vi "GetProbePlanCoordinates.vi"(1 "Probe Card Channels":i32=32) -> (0 "file path":string, 2 "OK?":bool, 3 "Array":T1(array[cluster]))   [LabVIEW 2019]
doc: "Utility to read probe plan from text file and generate respective coordinates in global variable."
uses:
  general_VIs/globals/QC_MeasurementSetup.vi
  ProbePlanParams.vi
  <vilib>/regexp/Match Regular Expression.xnode
panel:
  out "No. probe points":string
  in  "ProbePoints":T2
  out "String":string
  in  "Stop Button":bool
  in  "OK Button":bool
  in  "Region":u16(ring)
  out "Coordinates":string[][](table)
  # "ProbePlan Coordinates"
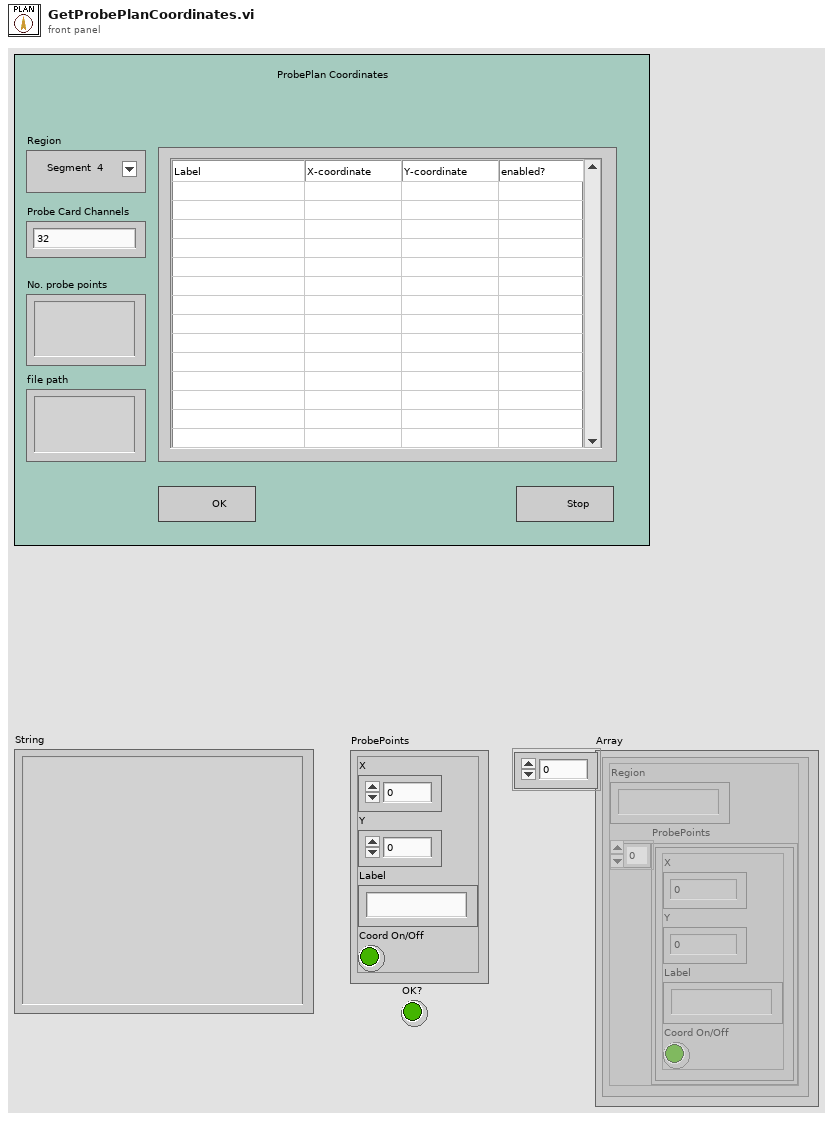
[diagram p1: front panel]
types:
  T1 = cluster{"Region":string, "ProbePoints":cluster{"X":dbl, "Y":dbl, "Label":string, "Coord On/Off":bool}[]}[]
  T2 = cluster{"X":dbl, "Y":dbl, "Label":string, "Coord On/Off":bool}
  T3 = cluster{"Region":string, "ProbePoints":cluster{"X":dbl, "Y":dbl, "Label":string, bool}[]}[]
  T4 = enum16{"open", "replace", "create", "open or create", "replace or create", "replace or create with confirmation"}
  T5 = cluster{"X":dbl, "Y":dbl, "Label":string, bool}[]
  T6 = cluster{"Bias Supply":refnum<class "SupplyControl.lvclass">, "SMU":refnum<class "SupplyControl.lvclass">, "LCR":refnum<class "LCRControl.lvclass">, "Probe Card Channels":i32, "Bias Voltage [V]":dbl, "First strip":i32, "Last strip":i32, "Base Voltage [V]":dbl, "Base Ramp Step [V]":dbl, "Base Ramp Interval [ms]":u32, "High Voltage [V]":dbl, "High Ramp Step [V]":dbl, "High Ramp Interval [ms]":u32, "AC frequency [Hz]":i32, "AC amplitude [V]":dbl, "RC Configuration":u16, "Single Needle":bool, "Temperature Readout":enum16{"Read Arduino", "Enter manually"}, "Arduino":refnum<class "ArduinoControl.lvclass">, "Fraction of good strips [%]":dbl, "ProbeStation":refnum<class "ProbeStationControl.lvclass">, "Switching":refnum<class "Switching.lvclass">, "Matrix used?":bool, "Matrix X Channels":cluster{"Bias Supply / SMU LO":i32, "Bias Supply / SMU HI":i32, "CV Box LO":i32, "CV Box HI":i32, "CV Box LO IN":i32, "CV Box HI IN":i32, "Volt meter LO":i32, "Volt meter HI":i32, "Mux1 C1":i32, "Mux1 C2":i32, "Mux2 C1":i32, "Mux2 C2":i32}, "Pinholes Y/N":bool, "Capacitance Y/N":bool, "Resistance Y/N":bool, "Bias Supply Name":string, "SMU Name":string, "LCR Name":string}
  T7 = cluster{"submatch 1":string, "ProbePoints":cluster{"X":dbl, "Y":dbl, "Label":string, bool}[]}
  T8 = cluster{"submatch 1":string, "ProbePoints":cluster{"X":dbl, "Y":dbl, "Label":string, bool}[]}[]
  T9 = cluster{"Region":string, "ProbePoints":cluster{"X":dbl, "Y":dbl, "Label":string, bool}[]}
  T10 = cluster{"X":dbl, "Y":dbl, "Label":string, "Coord On/Off":bool}[]
  T11 = cluster{"Region":string, cluster{"X":dbl, "Y":dbl, "Label":string, "Coord On/Off":bool}[]}
  T12 = cluster{"Strip Number OUT":i32, "X0":i32, "Y0":i32, "X1":i32, "Y1":i32, "Xref":dbl, "Yref":dbl, "ProbePlan type":u32, "Inner pads offset":ext, "Outer pads offset":ext, "l_inner":ext, "l_outer":ext, "strip numbering":u16, "Device Orientation":ext, "Stagger offset":i32, "Yoffset":dbl, "Strip pitch":dbl, "Fiducail separation":dbl, "Radius":ext, "Relative strip angles":dbl, "Probeplan description":string, "ProbePlan array":cluster{"Region":string, "ProbePoints":cluster{"X":dbl, "Y":dbl, "Label":string, "CardViable?":bool}[]}[], "Test ProbePoints":cluster{"Regions Enabled":bool[], "From index":u32[], "To index":u32[]}}
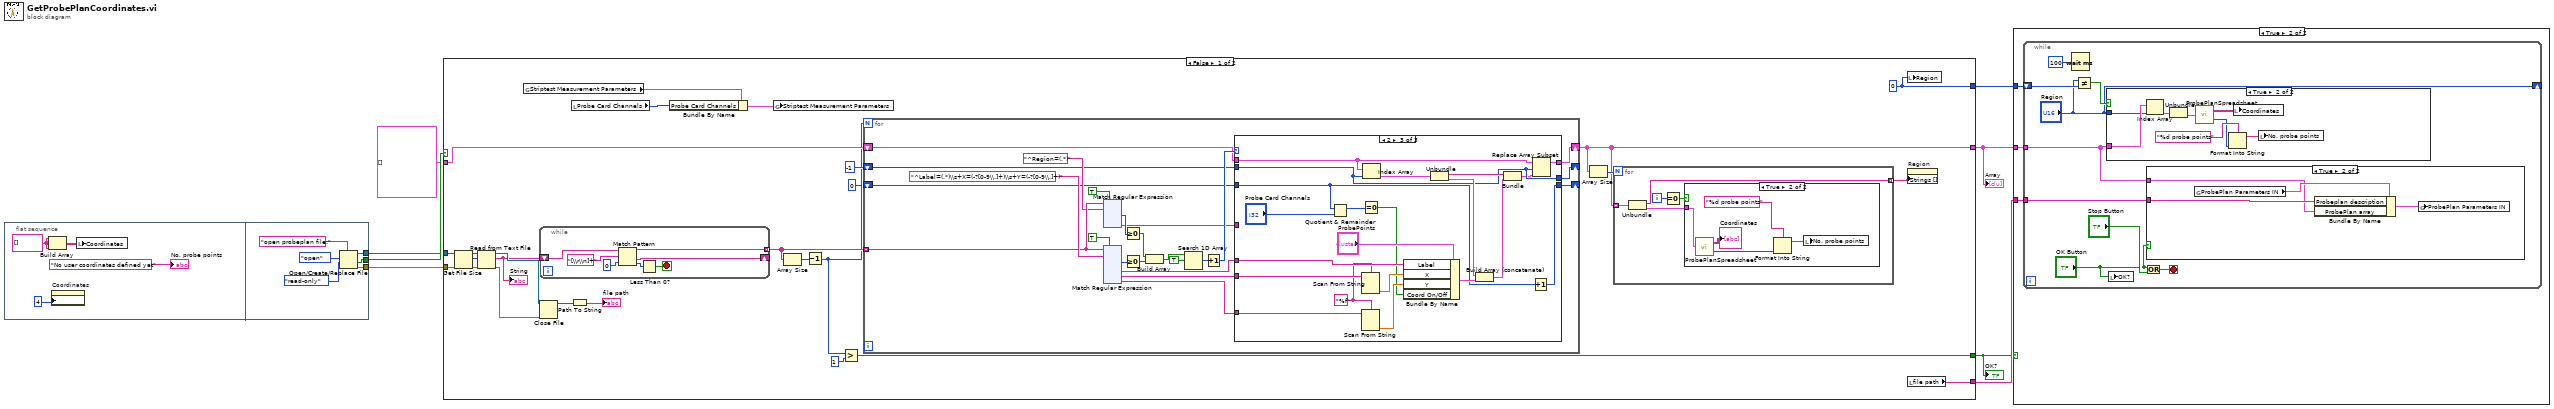
[diagram p0: block diagram]
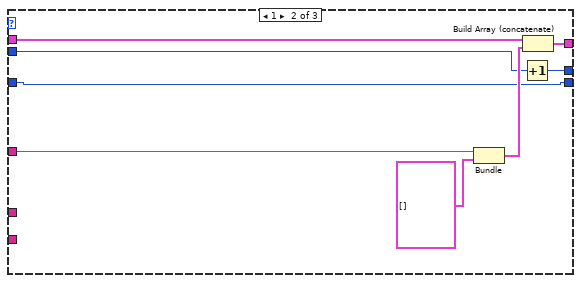
[diagram p7: hidden frame]
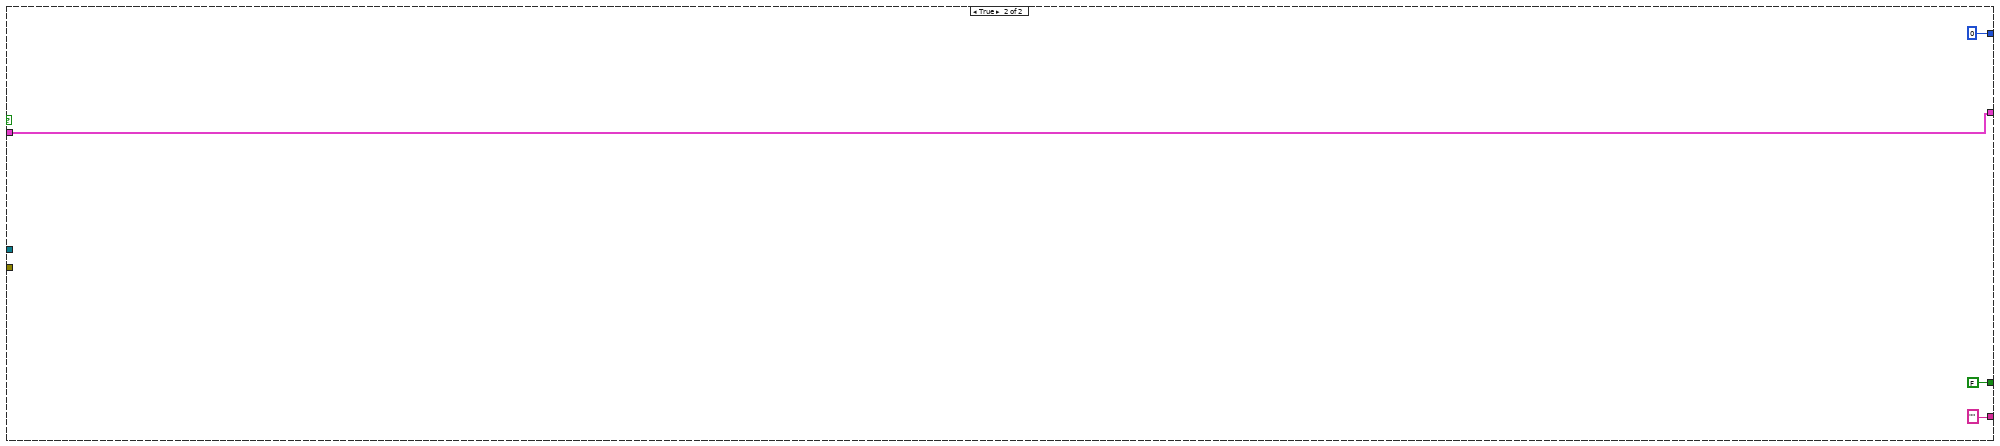
[diagram p8: hidden frame]
diagram:
  n1 = flat-sequence {
    tunnel: [w15] -> w8
    tunnel: [w14] -> w6
    tunnel: [w13] -> w7
    frame #0 {
      w12 = string[] []
      n2 = Build Array(w12, w12, w12) -> (w11:string[][])
      n3 = property on="Coordinates" class="Tbl (strict)"("Number of Columns"=4) -> ()  [unwired: 2 in, 2 out]
      n4 = local write "Coordinates"(w11) -> ()
      "No. probe points" <- "No user coordinates defined yet" ("String 2")
    }
    frame #1 {
      n5 = Open/Create/Replace File(prompt="open probeplan file:", operation (0:open)=T4."open", access (0:read/write)=enum16{"read/write", "read-only", "write-only"}."read-only") -> (refnum out=w13:refnum<file>, cancelled=w15:bool, error out=w14:errorcluster)  [unwired: 3 in]
    }
  }
  n6 = case shown="False" w8 {
    tunnel: T3 [] ("Array") -> [w31 w354]
    tunnel: w7 -> [w44 _]
    tunnel: w6 -> [w39 _]
    tunnel: [w29 w354] -> w4
    tunnel: [w28 0] -> w3
    tunnel: [w24 FALSE] -> w2
    tunnel: [w23 ""] -> w5
    frame False {
      w28 = 0
      n7 = Get File Size(file=w44, error in=w39) -> (refnum out=w43:refnum<file>, size (in bytes)=w38:i64, 0:w41:errorcluster)
      n8 = Read from Text File(file (use dialog)=w43, count=w38, error in=w41) -> (refnum out=w42:refnum<file>, text=w35:string, error out=w40:errorcluster)  [unwired: 1 in, 1 out]
      "String" <- w35
      n9 = global read "QC_MeasurementSetup.vi" "Striptest Measurement Parameters"() -> (w20:T6)
      n10 = while {
        shift-right: [w347] -> _
        shift-left: w35 -> [w350]
        tunnel: [w344] -> w33 mode=indexing
        stop <- w346 stop-if-true
        n11 = Match Pattern(string=w350, regular expression="[\\r\\n]+", offset (0)=0) -> (before substring=w344:string, after substring=w347:string, offset past match=w345:i32)  [unwired: 1 out]
        n12 = Less Than 0?(x=w345) -> (x < 0?=w346:bool)
      }
      n13 = Close File(refnum=w42, error in=w40) -> (path=w37:path)  [unwired: 1 out]
      n14 = Path To String(path=w37) -> (string=→"file path":string)
      n15 = local read "Probe Card Channels"() -> (w21:i32)
      n16 = Bundle By Name(cluster=w20, "Probe Card Channels"=w21) -> (w19:T6)
      n17 = global write "QC_MeasurementSetup.vi" "Striptest Measurement Parameters"(w19) -> ()
      n18 = Array Size(array=w33) -> (size(s)=w34:i32)
      n19 = Decrement(x=w34) -> (x-1=w25:i32)
      n20 = Greater?(x=w25, y=1) -> (0:w24:bool)
      n21 = for {
        N: w25 -> [_]
        tunnel: w33 -> [w71] mode=indexing
        shift-right: [w57] -> _
        shift-left: -1 -> [w58]
        shift-right: [w59] -> w29
        shift-left: w31 -> [w60]
        shift-right: [w56] -> _
        shift-left: 0 -> [w55]
        n22 = xnode "Match Regular Expression"("input string"=w71, "regular expression"="^Region=(.*)", "ignore case? (F)"=TRUE) -> ("offset past match"=w68:i32, "submatch 1"=w61:string)  [unwired: 3 in, 4 out]
        n23 = xnode "Match Regular Expression"("input string"=w71, "regular expression"="^Label=(.*)\\s+X=(-?[0-9\\.]+)\\s+Y=(-?[0-9\\.]+)", "ignore case? (F)"=TRUE) -> ("offset past match"=w74:i32, "submatch 1"=w75:string, "submatch 2"=w72:string, "submatch 3"=w73:string)  [unwired: 3 in, 4 out]
        n24 = Greater Or Equal To 0?(x=w68) -> (x >= 0?=w67:bool)
        n25 = Greater Or Equal To 0?(x=w74) -> (x >= 0?=w66:bool)
        n26 = Build Array(w67, w66) -> (w65:bool[])
        n27 = Search 1D Array(1D array=w65, element=TRUE) -> (index of element=w63:i32)  [unwired: 1 in]
        n28 = Increment(x=w63) -> (x+1=w62:i32)
        n29 = case shown="2" w62 {
          tunnel: w75 -> [_ _ w222]
          tunnel: w73 -> [_ _ w219]
          tunnel: w72 -> [_ _ w221]
          tunnel: w61 -> [_ w204 _]
          tunnel: w60 -> [w196 w202 w214]
          tunnel: [w196 w200 w212] -> w59
          tunnel: w58 -> [w195 w199 w215]
          tunnel: [w195 w198 w215] -> w57
          tunnel: [w194 w197 w206] -> w56
          tunnel: w55 -> [w194 w197 w205]
          frame 0, Default {
          }
          frame 1 {
            n30 = Bundle("submatch 1"=w204, "ProbePoints"=T5 []) -> (w201:T7)  [unwired: 1 in]
            n31 = Increment(x=w199) -> (x+1=w198:i32)
            n32 = Build Array (concatenate)(w202, w201) -> (w200:T8)
          }
          frame 2 {
            w218 = "%f" ("format string")
            n33 = Quotient & Remainder(x=w205, y="Probe Card Channels") -> (x-y*floor(x/y)=w209:i32)  [unwired: 1 out]
            n34 = Scan From String(format string=w218, input string=w221) -> (output 1=w220:dbl)  [unwired: 3 in, 3 out]
            n35 = Scan From String(format string=w218, input string=w219) -> (output 1=w217:dbl)  [unwired: 3 in, 3 out]
            n36 = Index Array(array=w214, index=w215) -> (element=w225:T9)
            n37 = Equal To 0?(x=w209) -> (x = 0?=w207:bool)
            n38 = Bundle By Name(cluster="ProbePoints", "Label"=w222, "X"=w220, "Y"=w217, "Coord On/Off"=w207) -> (w210:T2)
            n39 = Unbundle(w225) -> ("Region"=w224:string, "ProbePoints"=w223:T5)
            n40 = Build Array (concatenate)(w223, w210) -> (w216:T10)
            n41 = Bundle("Region"=w224, w216) -> (w213:T11)  [unwired: 1 in]
            n42 = Increment(x=w205) -> (x+1=w206:i32)
            n43 = Replace Array Subset(array=w214, new element=w213, index=w215) -> (w212:T3)
          }
        }
      }
      n44 = Array Size(array=w29) -> (size(s)=w30:i32)
      n45 = for {
        N: w30 -> [_]
        tunnel: w29 -> [w49] mode=indexing
        tunnel: [w48] -> w27 mode=indexing
        i -> [w46]
        n46 = Unbundle(w49) -> ("Region"=w48:string, "ProbePoints"=w47:T5)
        n47 = Equal To 0?(x=w46) -> (x = 0?=w45:bool)
        n48 = case shown="True" w45 {
          tunnel: w47 -> [_ w52]
          frame False {
          }
          frame True {
            n49 = call "ProbePlanSpreadsheet.vi"("ProbePoints"=w52) -> ("Coordinates"=→"Coordinates":string[][], "Number of ProbePoints"=w51:i32)
            n50 = Format Into String(format string="%d probe points", w51) -> (resulting string=w53:string)  [unwired: 2 in, 1 out]
            n51 = local write "No. probe points"(w53) -> ()
          }
        }
      }
      n52 = local write "Region"(w28) -> ()
      n53 = property on="Region" class="Ring (strict)"("Strings []"=w27) -> ()  [unwired: 2 in, 2 out]
      n54 = local read "file path"() -> (w23:string)
    }
    frame True {
    }
  }
  "Array" <- w4
  "OK?" <- w2
  n55 = case shown="True" w2 {
    tunnel: w3 -> [_ w357]
    tunnel: w4 -> [_ w356]
    tunnel: w5 -> [_ w355]
    frame False {
    }
    frame True {
      n56 = while {
        shift-right: ["Region"] -> _
        shift-left: w357 -> [w365]
        tunnel: w356 -> [w362]
        tunnel: w355 -> [w361]
        stop <- w366 stop-if-true
        n57 = Wait (ms)(milliseconds to wait=u32 100) -> ()  [unwired: 1 out]
        n58 = Not Equal?(x="Region", y=w365) -> (x != y?=w364:bool)
        n59 = case shown="True" w364 {
          tunnel: w362 -> [_ w378]
          tunnel: "Region" -> [_ w376]
          frame False {
          }
          frame True {
            n60 = Index Array(array=w378, index=w376) -> (element=w377:T9)
            n61 = Unbundle(w377) -> ("ProbePoints"=w373:T5)  [unwired: 1 out]
            n62 = call "ProbePlanSpreadsheet.vi"("ProbePoints"=w373) -> ("Coordinates"=w371:string[][], "Number of ProbePoints"=w372:i32)
            n63 = Format Into String(format string="%d probe points", w372) -> (resulting string=w375:string)  [unwired: 2 in, 1 out]
            n64 = local write "Coordinates"(w371) -> ()
            n65 = local write "No. probe points"(w375) -> ()
          }
        }
        n66 = local write "OK?"("OK Button") -> ()
        n67 = Or(x="OK Button", y="Stop Button") -> (x .or. y?=w366:bool)
        n68 = case shown="True" "OK Button" {
          tunnel: w362 -> [_ w367]
          tunnel: w361 -> [_ w368]
          frame False {
          }
          frame True {
            n69 = global read "ProbePlanParams.vi" "ProbePlan Parameters IN"() -> (w370:T12)
            n70 = Bundle By Name(cluster=w370, "Probeplan description"=w368, "ProbePlan array"=w367) -> (w369:T12)
            n71 = global write "ProbePlanParams.vi" "ProbePlan Parameters IN"(w369) -> ()
          }
        }
      }
    }
  }
